vi "Generate Public Member Icons.vi"(8 "error in (no error)":errorcluster, 11 "Icon Destination Path":path) -> (0 "error out":errorcluster)   [LabVIEW 2015]
uses:
  Device/Device.lvclass
  Window/Window.lvclass
  <vilib>/Utility/NIReport.llb/NI_ReportGenerationCore.lvlib
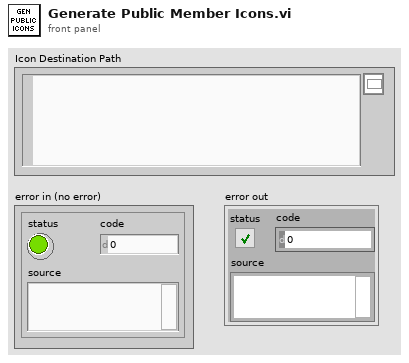
[diagram p1: front panel]
types:
  T1 = enum32{"invalid scope", "public", "private", "protected", "community"}
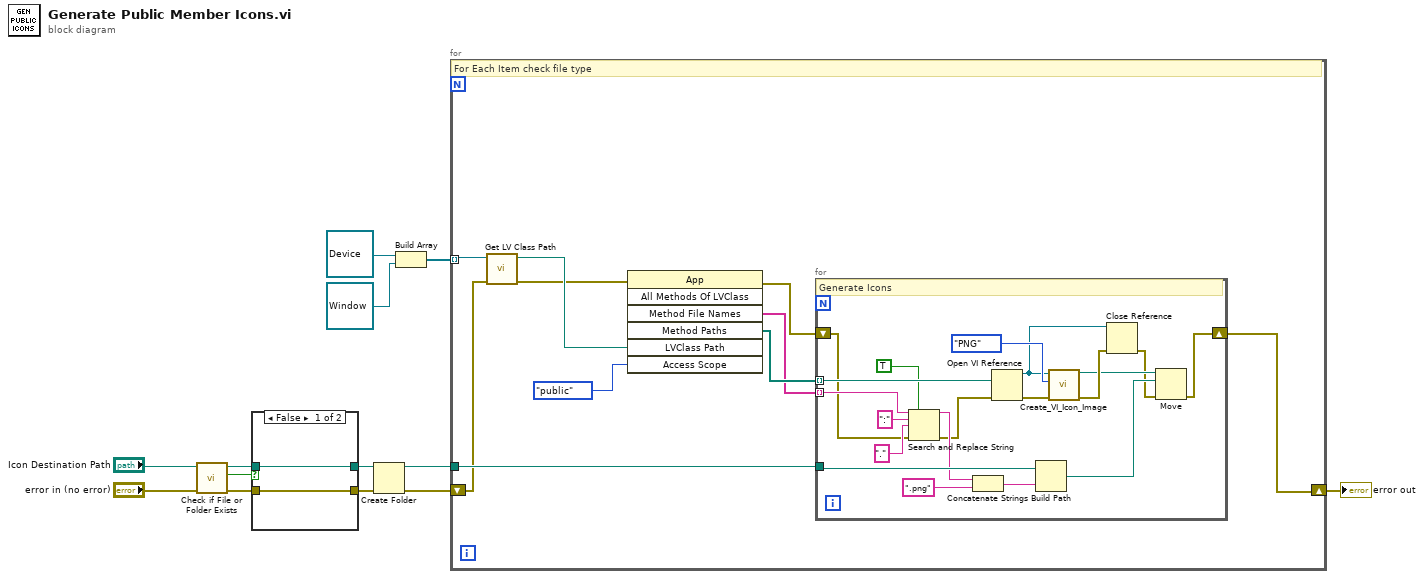
[diagram p0: block diagram]
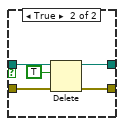
[diagram p2: hidden frame]
diagram:
  n1 = call <vilib>:"Check if File or Folder Exists.vi"("error in (no error)"="error in (no error)", "path"="Icon Destination Path") -> ("error out"=w10:errorcluster, "file or folder exists?"=w12:bool, "dup path"=w11:path)  [unwired: 7 in]
  n2 = case shown="False" w12 {
    tunnel: w11 -> [w15 w19]
    tunnel: w10 -> [w14 w20]
    tunnel: [w15 w17] -> w7
    tunnel: [w14 w16] -> w8
    frame False {
    }
    frame True {
      n3 = Delete(path (use dialog)=w19, entire hierarchy (F)=TRUE, error in=w20) -> (deleted path=w17:path, error out=w16:errorcluster)  [unwired: 2 in, 1 out]
    }
  }
  n4 = Create Folder(path (use dialog)=w7, error in=w8) -> (created path=w5:path, error out=w6:errorcluster)  [unwired: 1 in, 1 out]
  n5 = Build Array(refnum<class "Device.lvclass"> refnum ("IBEX Device.lvlib:Device.lvclass"), refnum<class "Window.lvclass"> refnum ("IBEX Device.lvlib:Window.lvclass")) -> (w1:refnum<class>[])
  n6 = for {
    shift-right: [w29] -> w4
    shift-left: w6 -> [w23]
    tunnel: w5 -> [w30]
    tunnel: w1 -> [w24] mode=indexing
    # "For Each Item check file type"
    n7 = call <vilib>:"Get LV Class Path.vi"("error in (no error)"=w23, "object"=w24) -> ("error out"=w21:errorcluster, "class path"=w22:path)  [unwired: 8 in]
    n8 = invoke class="App" method="All Methods Of LVClass"(error in=w21, "LVClass Path"=w22, "Access Scope"=T1."public") -> (error out=w26:errorcluster, "Method File Names"=w25:string[], "Method Paths"=w27:path[])  [unwired: 4 in, 4 out]
    n9 = for {
      tunnel: w30 -> [w46]
      shift-right: [w43] -> w29
      shift-left: w26 -> [w35]
      tunnel: w27 -> [w42] mode=indexing
      tunnel: w25 -> [w39] mode=indexing
      # "Generate Icons"
      n10 = Search and Replace String(replace all?=TRUE ("replace all? (F)"), input string=w39, search string=":", replace string="." ("replace string (\"\")"), error in=w35) -> (result string=w36:string, error out=w34:errorcluster)  [unwired: 3 in, 2 out]
      n11 = Concatenate Strings(w36, ".png" ("string")) -> (w32:string)
      n12 = Open VI Reference(vi path=w42, error in (no error)=w34) -> (vi reference=w40:refnum<vi>, error out=w41:errorcluster)  [unwired: 4 in]
      n13 = Build Path(base path=w46, name or relative path=w32) -> (appended path=w45:path)
      n14 = call <vilib>:"Create_VI_Icon_Image.vi"("error in (no error)"=w41, "Image Format (jpeg)"=enum32{"PNG", "JPEG", "GIF"}."PNG", "VI"=w40) -> ("error out"=w48:errorcluster, "Path to image"=w47:path)  [unwired: 7 in]
      n15 = Close Reference(reference=w40, error in (no error)=w48) -> (error out=w44:errorcluster)
      n16 = Move(source path=w47, error in=w44, 10:w45) -> (error out=w43:errorcluster)  [unwired: 2 in, 2 out]
    }
  }
  "error out" <- w4
